vi "ExecutePythonScript.vi"(8 "error in":errorcluster, 10 "Path to Python Script":string, 11 "Path to Python.exe":string) -> (0 "error out":errorcluster, 2 "array type (2D Dbl)":dbl[](array[numeric]), 3 "standard output":string)   [LabVIEW 2013, in "JCPython.lvclass"]
uses:
  JCPython.lvclass
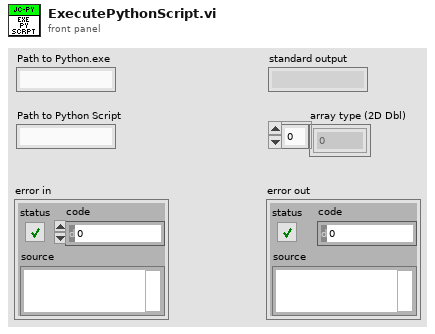
[diagram p1: front panel]
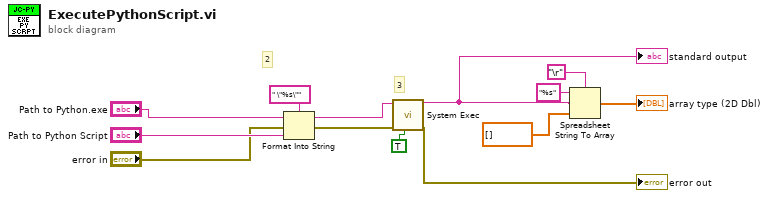
[diagram p0: block diagram]
diagram:
  # "3"
  # "2"
  n1 = Format Into String(format string=" \"%s\"", initial string="Path to Python.exe", error in="error in", "Path to Python Script") -> (resulting string=w10:string, error out=w8:errorcluster)
  n2 = call "System Exec.vi"("run minimized? (F)"=TRUE, "error in (no error)"=w8, "command line"=w10) -> ("error out"=→"error out":errorcluster, "standard output"=w5:string)  [unwired: 5 in, 2 out]
  "standard output" <- w5
  n3 = Spreadsheet String To Array(delimiter (Tab)="\r", format string="%s", spreadsheet string=w5, array type (2D Dbl)=dbl[] []) -> (array=→"array type (2D Dbl)":dbl[])
